vi "clear.vi"(8 "error in (no error)":errorcluster, 11 "Image in":refnum<class "Image.lvclass">) -> (0 "error out":errorcluster, 3 "Image out":refnum<class "Image.lvclass">)   [LabVIEW 2010, in "Image.lvclass"]
uses:
  Image.lvclass
  storage_mode.ctl
  ErrorController/ErrorController/class_data.vi
  <vilib>/vision/NI_Vision_Development_Module.lvlib
  ErrorController/ErrorController/ErrorController.lvclass
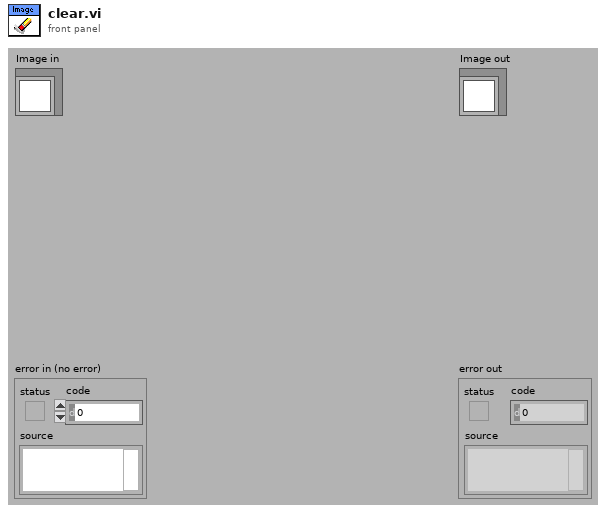
[diagram p1: front panel]
types:
  T1 = typedef "Image.lvclass/storage_mode.ctl" = enum16{"RAM", "disk"}
  T2 = typedef "IMAQ Image.ctl" = refnum<image>
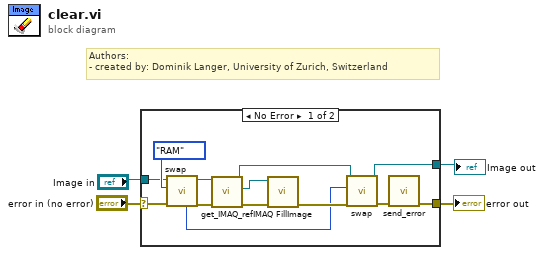
[diagram p0: block diagram]
diagram:
  # "Authors: \n- created by: Dominik Langer, University of Zurich, Switzerland"
  n1 = case shown="No Error" "error in (no error)" {
    selector: "error in (no error)" -> [w17 w19]
    tunnel: [w5 w19] -> w3
    tunnel: "Image in" -> [w8 w18]
    tunnel: [w10 w18] -> w1
    frame No Error {
      n2 = call-dynamic "swap.vi"("error in (no error)"=w17, "storage type target"=storage_mode."RAM", "Image in"=w8) -> ("error out"=w16:errorcluster, "Image out"=w7:refnum<class "Image.lvclass">, "previous storage mode"=w12:T1)  [unwired: 6 out]
      n3 = call-dynamic "get_IMAQ_ref.vi"("error in (no error)"=w16, "Image.lvclass in"=w7) -> ("error out"=w14:errorcluster, "Image"=w15:T2, "Image.lvclass out"=w11:refnum<class "Image.lvclass">)  [unwired: 7 out]
      n4 = call "IMAQ FillImage"("error in (no error)"=w14, "Image"=w15) -> ("error out"=w13:errorcluster)  [unwired: 5 in, 4 out]
      n5 = call-dynamic "swap.vi"("error in (no error)"=w13, "storage type target"=w12, "Image in"=w11) -> ("error out"=w6:errorcluster, "Image out"=w10:refnum<class "Image.lvclass">)  [unwired: 7 out]
      n6 = call "send_error.vi"("error in (no error)"=w6) -> ("error out"=w5:errorcluster)  [unwired: 10 in]
    }
    frame Error {
    }
  }
  "error out" <- w3
  "Image out" <- w1
